vi "Forward Kinematics.vi"(8 "error in (no error)":errorcluster, 10 "motor angles":dbl[](array[numeric])=[0.0, 0.0, 0.0, 0.0, 0.0, 0.0, 0.0], 11 "Finger in":refnum<class "Finger.lvclass">) -> (0 "error out":errorcluster, 1 "joint angles":dbl[](array[numeric]), 2 "T":T1=[[1.0, 0.0, 0.0, 0.0], [0.0, 1.0, 0.0, 0.0], [0.0, 0.0, 1.0, 0.0], [0.0, 0.0, 0.0, 1.0]], 3 "Finger out":refnum<class "Finger.lvclass">)   [LabVIEW 2011, in "Finger.lvclass"]
uses:
  Finger.lvclass
  <vilib>/Analysis/Matrix/Datatypes/RealMatrix.ctl
  Finger.lvclass/Finger.ctl
  <vilib>/Analysis/Matrix/Numeric/Multiply/Multiply - RM,RM.vi
  <vilib>/Analysis/Matrix/Numeric/Conversions/Array To Matrix - RA2.vi
  <vilib>/Analysis/Matrix/Numeric/Conversions/Array To Matrix - RA.vi
  <vilib>/Analysis/Matrix/Numeric/Multiply/Multiply - R,RM.vi
  <vilib>/Analysis/Matrix/Numeric/Multiply/Multiply - RM,R.vi
  <vilib>/Analysis/Matrix/Numeric/Add/Add - RM,RM.vi
  <vilib>/Analysis/Matrix/Numeric/Subtract/Subtract - RM,RM.vi
  <vilib>/Analysis/Matrix/NI_Matrix.lvlib
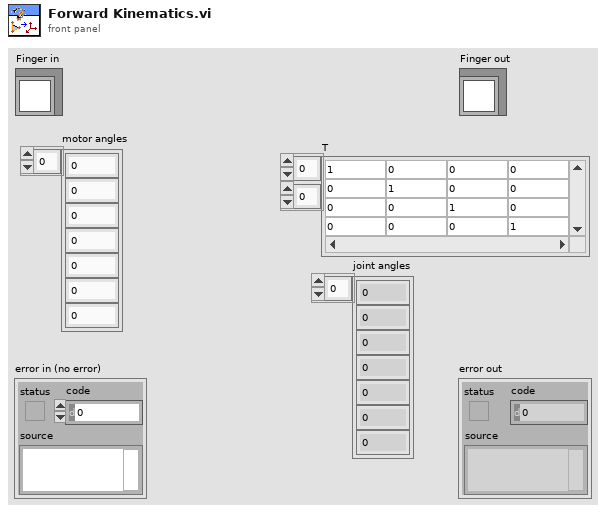
[diagram p1: front panel]
types:
  T1 = typedef "NI_Matrix.lvlib/RealMatrix.ctl" = dbl[][]
  T2 = typedef "5-bar Side.ctl" = enum16{"Left", "Right"}
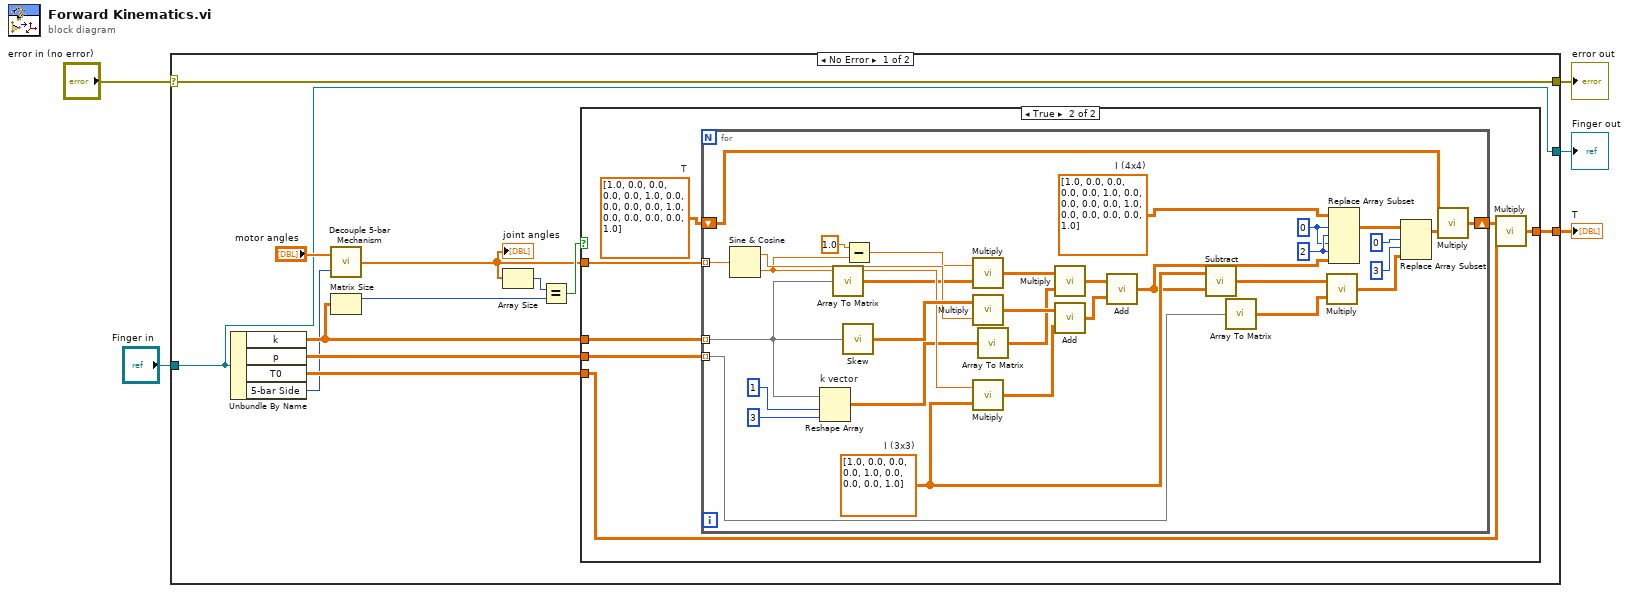
[diagram p0: block diagram]
diagram:
  n1 = case shown="No Error" "error in (no error)" {
    selector: "error in (no error)" -> [w17 w58]
    tunnel: [w17 w58] -> w4
    tunnel: [w7 w57] -> w2
    tunnel: "Finger in" -> [w7 w57]
    tunnel: [w11 _] -> w1
    frame No Error {
      n2 = Unbundle By Name(w7) -> ("k"=w16:T1, "p"=w15:T1, "T0"=w14:T1, "5-bar Side"=w6:T2)
      n3 = call "Decouple 5-bar Mechanism.vi"("5-bar Side"=w6, "motors angles"="motor angles") -> ("joint angles"=w9:dbl[])  [unwired: 1 in]
      "joint angles" <- w9
      n4 = Matrix Size(0:w16) -> (1:w12:i32)  [unwired: 1 out]
      n5 = Array Size(array=w9) -> (size(s)=w13:i32)
      n6 = Equal?(x=w13, y=w12) -> (x = y?=w10:bool)
      n7 = case shown="True" w10 {
        tunnel: w9 -> [_ w24]
        tunnel: w15 -> [_ w23]
        tunnel: w16 -> [_ w22]
        tunnel: [_ w19] -> w11
        tunnel: w14 -> [_ w18]
        frame False {
        }
        frame True {
          w21 = T1 [[1.0, 0.0, 0.0, 0.0], [0.0, 1.0, 0.0, 0.0], [0.0, 0.0, 1.0, 0.0], [0.0, 0.0, 0.0, 1.0]]  # T
          n8 = for {
            tunnel: w24 -> [w56] mode=indexing
            tunnel: w23 -> [w31] mode=indexing
            tunnel: w22 -> [w34] mode=indexing
            shift-right: [w38] -> w20
            shift-left: w21 -> [w39]
            w44 = 2 ("row N")
            w43 = 0 ("row 1")
            w45 = T1 [[1.0, 0.0, 0.0, 0.0], [0.0, 1.0, 0.0, 0.0], [0.0, 0.0, 1.0, 0.0], [0.0, 0.0, 0.0, 1.0]]  # I (4x4)
            w42 = T1 [[1.0, 0.0, 0.0], [0.0, 1.0, 0.0], [0.0, 0.0, 1.0]]  # I (3x3)
            n9 = Sine & Cosine(0:w56) -> (1:w54:dbl, 2:w50:dbl)
            n10 = Reshape Array "k vector"(w34, 1 ("dimension size"), 3 ("dimension size")) -> (w32:dbl[][])
            n11 = call-poly <vilib>:"Array To Matrix.vi"("Real 1D Array"=w34) -> ("Real Matrix (Column Vector)"=w37:T1)
            n12 = call "Skew.vi"("k"=w34) -> ("M"=w55:T1)
            n13 = Subtract(x=1.0, y=w50) -> (x-y=w49:dbl)
            n14 = call-poly <vilib>:"Multiply.vi"("Real Matrix A"=w37, "Real Scalar c"=w49) -> ("c * A"=w48:T1)
            n15 = call-poly <vilib>:"Multiply.vi"("Real Scalar c"=w54, "Real Matrix A"=w55) -> ("A * c"=w52:T1)
            n16 = call-poly <vilib>:"Multiply.vi"("Real Matrix A"=w42, "Real Scalar c"=w50) -> ("c * A"=w53:T1)
            n17 = call-poly <vilib>:"Array To Matrix.vi"("Real 2D Array"=w32) -> ("Real Matrix"=w33:T1)
            n18 = call-poly <vilib>:"Multiply.vi"("Real Matrix B"=w33, "Real Matrix A"=w48) -> ("A * B"=w46:T1)
            n19 = call-poly <vilib>:"Add.vi"("Real Matrix B"=w53, "Real Matrix A"=w52) -> ("A + B"=w47:T1)
            n20 = call-poly <vilib>:"Add.vi"("Real Matrix B"=w47, "Real Matrix A"=w46) -> ("A + B"=w41:T1)
            n21 = call-poly <vilib>:"Subtract.vi"("Real Matrix B"=w41, "Real Matrix A"=w42) -> ("A - B"=w40:T1)
            n22 = call-poly <vilib>:"Array To Matrix.vi"("Real 1D Array"=w31) -> ("Real Matrix (Column Vector)"=w30:T1)
            n23 = call-poly <vilib>:"Multiply.vi"("Real Matrix B"=w30, "Real Matrix A"=w40) -> ("A * B"=w27:T1)
            n24 = Replace Array Subset(array=w45, new element=w41, index (dim 0)=w43, index (dim 1)=w44, index (dim 2)=w43, index (dim 3)=w44) -> (w29:T1)
            n25 = Replace Array Subset(array=w29, new element=w27, index (row)=0 ("disabled index (row)"), index (col)=3 ("disabled index (col)")) -> (w28:T1)
            n26 = call-poly <vilib>:"Multiply.vi"("Real Matrix B"=w28, "Real Matrix A"=w39) -> ("A * B"=w38:T1)
          }
          n27 = call-poly <vilib>:"Multiply.vi"("Real Matrix B"=w18, "Real Matrix A"=w20) -> ("A * B"=w19:T1)
        }
      }
    }
    frame Error {
    }
  }
  "error out" <- w4
  "Finger out" <- w2
  "T" <- w1
